vi "UpdateValues.vi"(8 "error in (no error)":errorcluster, 10 "Path":path, 11 "ReportList in":refnum<class "ReportList.lvclass">) -> (0 "error out":errorcluster, 3 "ReportList out":refnum<class "ReportList.lvclass">)   [LabVIEW 2015, in "ReportList.lvclass"]
uses:
  ReportList.lvclass
  _list/List.lvclass/List.ctl
  <vilib>/Utility/file.llb/Read Delimited Spreadsheet (string).vi
  _list/List.lvclass
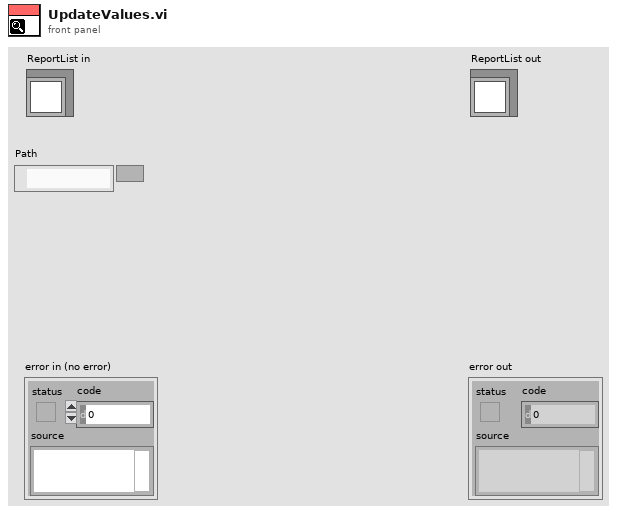
[diagram p1: front panel]
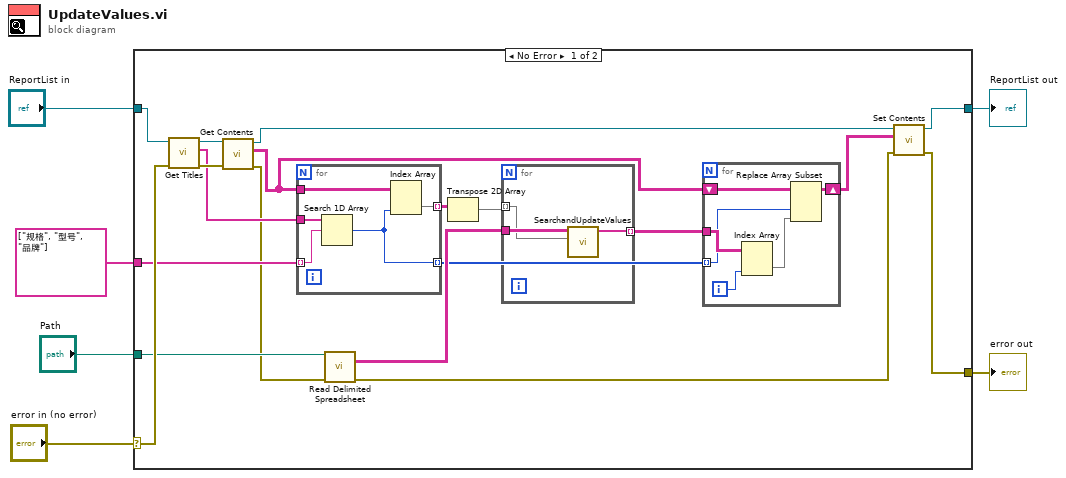
[diagram p0: block diagram]
diagram:
  n1 = case shown="No Error" "error in (no error)" {
    selector: "error in (no error)" -> [w24 w41]
    tunnel: [w11 w41] -> w5
    tunnel: [w10 w40] -> w3
    tunnel: "ReportList in" -> [w25 w40]
    tunnel: string[] ["规格", "型号", "品牌"] -> [w20 _]
    tunnel: "Path" -> [w19 _]
    frame No Error {
      n2 = call "Get Titles.vi"("error in (no error)"=w24, "List in"=w25) -> ("error out"=w22:errorcluster, "Titles"=w21:string[], "List out"=w23:refnum<class "ReportList.lvclass">)  [unwired: 7 in]
      n3 = call "Get Contents.vi"("error in (no error)"=w22, "List in"=w23) -> ("error out"=w13:errorcluster, "Contents"=w17:string[][], "List out"=w15:refnum<class "ReportList.lvclass">)  [unwired: 7 in]
      n4 = for {
        tunnel: w21 -> [w39]
        tunnel: w20 -> [w38] mode=indexing
        tunnel: w17 -> [w37]
        tunnel: [w36] -> w8 mode=indexing
        tunnel: [w35] -> w16 mode=indexing
        n5 = Search 1D Array(1D array=w39, element=w38) -> (index of element=w35:i32)  [unwired: 1 in]
        n6 = Index Array(array=w37, index (col)=w35) -> (element=w36:string[])  [unwired: 1 in]
      }
      n7 = call-poly <vilib>:"Read Delimited Spreadsheet.vi"("file path (dialog if empty)"=w19, "error in (no error)"=w13) -> ("all rows"=w18:string[][], "error out"=w12:errorcluster)  [unwired: 8 in, 4 out]
      n8 = Transpose 2D Array(2D array=w8) -> (transposed array=w7:string[][])
      n9 = for {
        tunnel: w7 -> [w33] mode=indexing
        tunnel: w18 -> [w34]
        tunnel: [w32] -> w9 mode=indexing
        n10 = call "SearchandUpdateValues.vi"("Contents"=w33, "Rules"=w34) -> ("New Contents"=w32:string[])  [unwired: 9 in]
      }
      n11 = for {
        tunnel: w16 -> [w26] mode=indexing
        tunnel: w9 -> [w30]
        shift-right: [w27] -> w14
        shift-left: w17 -> [w31]
        i -> [w28]
        n12 = Index Array(array=w30, index (col)=w28) -> (element=w29:string[])  [unwired: 1 in]
        n13 = Replace Array Subset(array=w31, new element=w29, index (col)=w26) -> (w27:string[][])  [unwired: 1 in]
      }
      n14 = call "Set Contents.vi"("error in (no error)"=w12, "Contents"=w14, "List in"=w15) -> ("error out"=w11:errorcluster, "List out"=w10:refnum<class "ReportList.lvclass">)  [unwired: 7 in]
    }
    frame Error {
    }
  }
  "error out" <- w5
  "ReportList out" <- w3
